vi "test Loopback.vi"(8 "error in":errorcluster, 11 "TestCase in":refnum<class "SingleCore.lvclass">) -> (0 "error out":errorcluster, 3 "TestCase out":refnum<class "SingleCore.lvclass">)   [LabVIEW 2020, in "SingleCore.lvclass"]
uses:
  SingleCore.lvclass
  C:/Users/Administrator/Git/niveristand-custom-device-testing-tools/VeriStandTestCase/VeriStandTestCase.lvclass
  4b06c685-66bb-4135-9ad1-d89a50a95502.vi
  <vilib>/numeric/Random Number (Range) I64.vi
  4cc353ea-8eb2-4b69-8f0e-bf7f0ec9a5d6.vi
  <vilib>/numeric/sub_Random U32.vi
  <vilib>/NI VeriStand/Execution/Workspace/NI VeriStand - Set Multiple Channel Values.vi
  <vilib>/NI VeriStand/Execution/Workspace/NI VeriStand - Get Multiple Channel Values.vi
  <vilib>/addons/_JKI Toolkits/VI Tester/TestCase.llb/TestCase.lvclass
  niveristand-custom-device-testing-tools/VeriStandTestCase/VeriStandTestCase.lvclass
  <vilib>/NI VeriStand/Execution/Workspace/NI_VS Workspace ExecutionAPI.lvlib
  C:/Program Files (x86)/National Instruments/LabVIEW 2020/vi.lib/addons/_JKI Toolkits/VI Tester/TestCase.llb/TestCase.lvclass
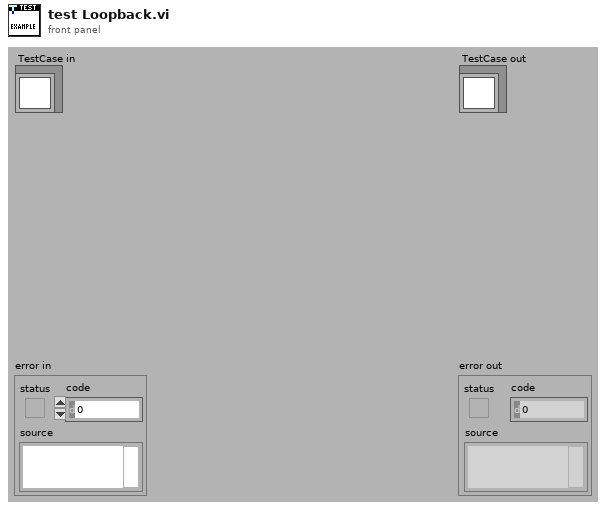
[diagram p1: front panel]
types:
  T1 = typedef "NI_VS Workspace ExecutionAPI.lvlib/WorkspaceAPI.ctl" = refnum<k24>
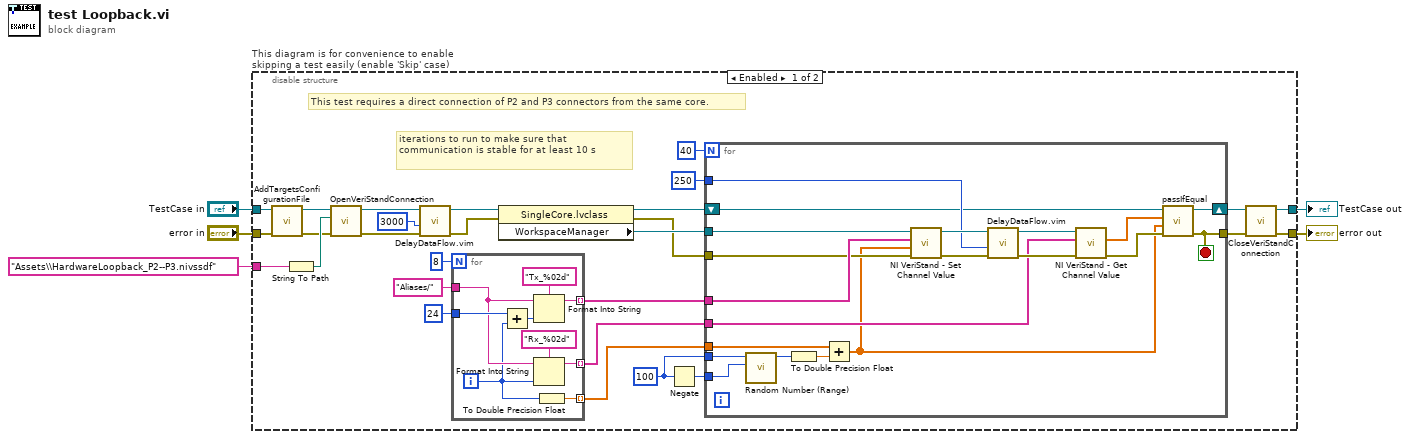
[diagram p0: block diagram]
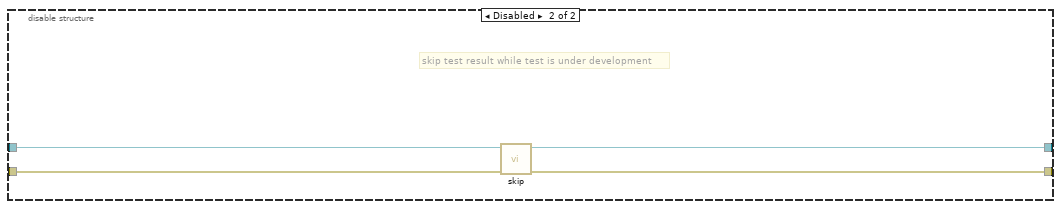
[diagram p2: hidden frame]
diagram:
  n1 = disable-structure "This diagram is for convenience to enable skipping a test easily (enable 'Skip' case)" shown="Enabled" {
    disable-tunnel: "TestCase in" -> [w32 w64]
    disable-tunnel: [w22 w62] -> w2
    disable-tunnel: [w21 w63] -> w4
    disable-tunnel: "error in" -> [w31 w61]
    disable-tunnel: "Assets\\HardwareLoopback_P2--P3.nivssdf" ("Channel") -> [w23 _]
    frame Enabled {
      w16 = i64 100 ("upper bound (100)")
      # "This test requires a direct connection of P2 and P3 connectors from the same core."
      # "iterations to run to make sure that communication is stable for at least 10 s"
      n2 = call "AddTargetsConfigurationFile.vi"("error in (no error)"=w31, "VeriStandTestCase in"=w32) -> ("error out"=w24:errorcluster, "VeriStandTestCase out"=w25:refnum<class "SingleCore.lvclass">)  [unwired: 8 in]
      n3 = String To Path(string=w23) -> (path=w26:path)
      n4 = call-dynamic "OpenVeriStandConnection.vi"("error in (no error)"=w24, "System Definition File"=w26, "VeriStand Test Case in"=w25) -> ("error out"=w28:errorcluster, "VeriStand Test Case out"=w30:refnum<class "SingleCore.lvclass">)  [unwired: 6 in, 1 out]
      n5 = call "DelayDataFlow.vim"("value in"=w28, "milliseconds to wait"=u32 3000) -> ("value out"=w27:errorcluster)  [unwired: 2 in, 1 out]
      n6 = for {
        N: 8 -> [_]
        tunnel: 24 ("x") -> [w60]
        tunnel: "Aliases/" ("Channel") -> [w56]
        tunnel: [w55] -> w14 mode=indexing
        tunnel: [w53] -> w9 mode=indexing
        tunnel: [w52] -> w17 mode=indexing
        i -> [w54]
        n7 = Add(x=w60, y=w54) -> (x+y=w57:i32)
        n8 = Format Into String(format string="Tx_%02d", initial string=w56, w57) -> (resulting string=w55:string)  [unwired: 1 in, 1 out]
        n9 = Format Into String(format string="Rx_%02d", initial string=w56, w54) -> (resulting string=w53:string)  [unwired: 1 in, 1 out]
        n10 = To Double Precision Float(number=w54) -> (double precision float=w52:dbl)
      }
      n11 = property class="SingleCore.lvclass"(reference=w30, error in=w27) -> (reference out=w8:refnum<class "SingleCore.lvclass">, error out=w10:errorcluster, "WorkspaceManager"=w13:T1)
      n12 = Negate(x=w16) -> (-x=w15:i64)
      n13 = for {
        N: 40 -> [_]
        tunnel: w17 -> [w46]
        tunnel: w16 -> [w45]
        tunnel: w15 -> [w44]
        tunnel: w14 -> [w43]
        tunnel: w13 -> [w42]
        tunnel: u32 250 ("milliseconds to wait") -> [w41]
        tunnel: w10 -> [w40]
        tunnel: w9 -> [w39]
        shift-right: [w36] -> w7
        shift-left: w8 -> [w37]
        tunnel: [w33] -> w6
        stop <- w33 stop-if-true
        n14 = call-poly <vilib>:"Random Number (Range).vi"("lower bound (-100)"=w44, "upper bound (100)"=w45) -> ("number"=w48:i64)  [unwired: 9 in]
        n15 = To Double Precision Float(number=w48) -> (double precision float=w47:dbl)
        n16 = Add(x=w46, y=w47) -> (x+y=w34:dbl[])
        n17 = call-poly <vilib>:"NI VeriStand - Set Channel Value.vi"("error in (no error)"=w40, "Values"=w34, "Channels"=w43, "WorkspaceManager in"=w42) -> ("error out"=w50:errorcluster, "WorkspaceManager out"=w49:T1)  [unwired: 6 in]
        n18 = call "DelayDataFlow.vim"("value in"=w50, "milliseconds to wait"=w41) -> ("value out"=w51:errorcluster)  [unwired: 2 in, 1 out]
        n19 = call-poly <vilib>:"NI VeriStand - Get Channel Value.vi"("error in (no error)"=w51, "Channels"=w39, "WorkspaceManager in"=w49) -> ("error out"=w38:errorcluster, "Values"=w35:dbl[])  [unwired: 6 in, 1 out]
        n20 = call-dynamic "passIfEqual.vi"("error in (no error)"=w38, "y"=w34, "x"=w35, "TestCase in"=w37) -> ("error out"=w33:errorcluster, "TestCase out"=w36:refnum<class "SingleCore.lvclass">)  [unwired: 6 in]
      }
      n21 = call-dynamic "CloseVeriStandConnection.vi"("error in (no error)"=w6, "VeriStand Test Case in"=w7) -> ("error out"=w21:errorcluster, "VeriStand Test Case out"=w22:refnum<class "SingleCore.lvclass">)  [unwired: 8 in]
    }
    frame Disabled {
      # "skip test result while test is under development"
      n22 = call <vilib>:"skip.vi"("error in (no error)"=w61, "TestCase in"=w64) -> ("error out"=w63:errorcluster, "TestCase out"=w62:refnum<class "SingleCore.lvclass">)  [unwired: 8 in]
    }
  }
  "error out" <- w4
  "TestCase out" <- w2
